vi "RSZVB Set Time Domain Transformation Type.vi"(8 "error in (no error)":errorcluster {"code" format="%.0x"}, 9 "Transformation Type (0: Band Pass Impulse)":i32(ring) items=["Band Pass Impulse", "Low Pass Impulse", "Low Pass Step"], 10 "Channel (Trace) (1)":i32=1, 11 "VISA session":refnum<visa-resource-name>) -> (0 "error out":errorcluster {"code" format="%.0x"}, 3 "dup VISA session":refnum<visa-resource-name>)   [LabVIEW 2011]
doc: "This VI defines time domain transformation type.\n\nRemote-control command(s):\nCALCulate<Ch/Tr>:TRANsform:TIME[:TYPE] BPASs | LPASs\nCALCulate<Ch/Tr>:TRANsform:TIME:STIMulus STEP | IMPulse"
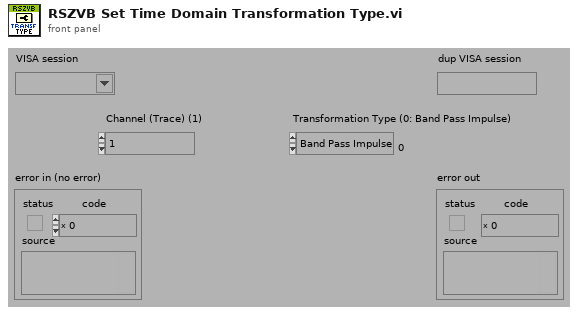
[diagram p1: front panel]
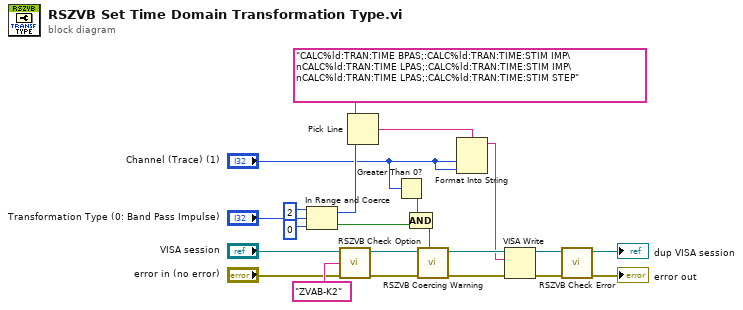
[diagram p0: block diagram]
diagram:
  n1 = In Range and Coerce(upper limit=2, x="Transformation Type (0: Band Pass Impulse)", lower limit=0) -> (coerced(x)=w11:i32, In Range?=w14:bool)
  n2 = call "RSZVB Check Option.vi"("error in (no error)"="error in (no error)", "Options"="ZVAB-K2", "VISA session"="VISA session") -> ("error out"=w10:errorcluster, "dup VISA session"=w9:refnum<visa-resource-name>)  [unwired: 7 in]
  n3 = Pick Line(multi-line string="CALC%ld:TRAN:TIME BPAS;:CALC%ld:TRAN:TIME:STIM IMP\nCALC%ld:TRAN:TIME LPAS;:CALC%ld:TRAN:TIME:STIM IMP\nCALC%ld:TRAN:TIME LPAS;:CALC%ld:TRAN:TIME:STIM STEP", line index=w11) -> (output string=w1:string)  [unwired: 1 in]
  n4 = Greater Than 0?(x="Channel (Trace) (1)") -> (x > 0?=w13:bool)
  n5 = Compound Arithmetic op=AND(w13, w14) -> (w12:bool)
  n6 = call "RSZVB Coercing Warning.vi"("In Range?"=w12, "error in (no error)"=w10, "VISA session"=w9) -> ("error out"=w21:errorcluster, "dup VISA session"=w22:refnum<visa-resource-name>)  [unwired: 7 in]
  n7 = Format Into String(format string=w1, "Channel (Trace) (1)", "Channel (Trace) (1)") -> (resulting string=w18:string)  [unwired: 2 in, 1 out]
  n8 = VISA Write(VISA resource name=w22, write buffer=w18, error in (no error)=w21) -> (VISA resource name out=w19:refnum<visa-resource-name>, error out=w20:errorcluster)  [unwired: 1 out]
  n9 = call "RSZVB Check Error.vi"("error in (no error)"=w20, "VISA session"=w19) -> ("error out"=→"error out":errorcluster, "dup VISA session"=→"dup VISA session":refnum<visa-resource-name>)  [unwired: 8 in]
